vi "Plot Upper & Lower CI Plots.vi"(0 "Y Array":dbl[](array[numeric]), 1 "XY Graph Ref":refnum<vi>, 2 "VI in":refnum<vi>, 3 "Additional LM Data":variant, 5 "X Array":dbl[](array[numeric]), 9 "Weight Array":dbl[](array[numeric]), 11 "error in (no error)":errorcluster, 12 "best fit parameters":dbl[](array[numeric]), 13 "Fitted Plot Name":string, 14 "confidence level (0.68)":dbl=0.68 format="%#_13g") -> (15 "error out":errorcluster)   [LabVIEW 2021, in "Fits.lvlib"]
doc: "Computes the upper and lower confidence interval plots and displays them in the XY Graph."
uses:
  Fits.lvlib
  Graphs/Single Plot Style 2.ctl
  Graphs/Graphs.lvlib
  AlliGator/Decay Analysis/Decay Fit/AlliGator Decay Fit.lvlib
  Graphs/XY Graph/XY Graph Add-Ons.lvlib
panel:
  # "see the License on the block diagram (Ctrl+E or Window:Show Block Diagram)"
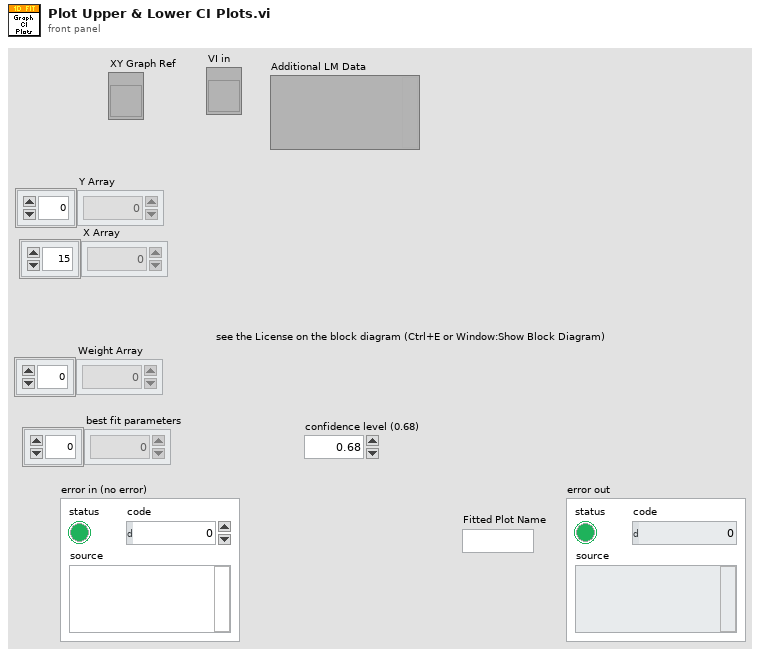
[diagram p1: front panel]
types:
  T1 = typedef "Graphs.lvlib/Single Plot Style 2.ctl" = cluster{"Plot Style":enum16{"unchanged", "Line", "Symbol", "Line + Symbol", "Histogram", "Histogram + Symbol"}, "Histogram Type":enum16{"unchanged", "Left Bound", "Center", "Right Bound"}, "Line Tickness":enum16{"unchanged", "Thin", "1 pixel", "2 pixel", "3 pixel", "4 pixel", "5 pixel"}, "Line Style":enum16{"unchanged", "Plain", "Long Dash", "Short Dash", "Long-Short Dash", "Long-Short-Short Dash"}, "Point Style":enum16{"unchanged", "None", "Empty Circle", "Filled Circle", "Thick Circle", "Dotted Circle", "Empty Square", "Filled Square", "Thick Square", "Dotted Square", "Small Filled Square", "Dot", "Cross", "Tiny Cross", "Large X", "Small x", "Diamond", "Small Empty Square"}, "Line Color":u32, "Line Color defined?":bool, "Point Color":u32, "Point Color defined?":bool, "Anti-aliased":bool}
  T2 = typedef "XY Graph Add-Ons.lvlib/XY Graph Plot Data.ctl" = cluster{"X Array":dbl[], "Y Array":dbl[]}
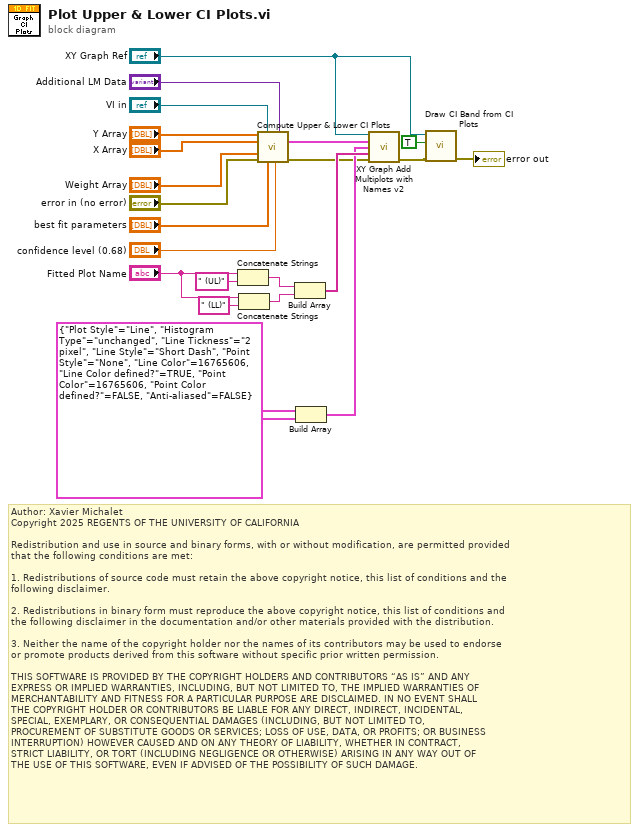
[diagram p0: block diagram]
diagram:
  w15 = T1 {"Plot Style"=enum."Line", "Histogram Type"=enum."unchanged", "Line Tickness"=enum."2 pixel", "Line Style"=enum."Short Dash", "Point Style"=enum."None", "Line Color"=16765606, "Line Color defined?"=TRUE, "Point Color"=16765606, "Point Color defined?"=FALSE, "Anti-aliased"=FALSE} ("Plot Style Array")
  # "Author: Xavier Michalet\nCopyright 2025 REGENTS OF THE UNIVERSITY OF CALIFORNIA\n\nRedistribution and use in source and binary forms, with or without modification, are permitted provided\nthat the following conditions are met:\n\n1. Redistributions of source code must retain the above copyright notice, this list of conditions and the\nfollowing disclaimer.\n\n2. Redistributions in binary form must reproduce the above copyright notice, this list of conditions and\nthe following disclaimer in the documentation and/or other materials provided with the distribution.\n\n3. Neither the name of the copyright holder nor the names of its contributors may be used to endorse \nor promote products derived from this software without specific prior written permission.\n\nTHIS SOFTWARE IS PROVIDED BY THE COPYRIGHT HOLDERS AND CONTRIBUTORS “AS IS” AND ANY \nEXPRESS OR IMPLIED WARRANTIES, INCLUDING, BUT NOT LIMITED TO, THE IMPLIED WARRANTIES OF\nMERCHANTABILITY AND FITNESS FOR A PARTICULAR PURPOSE ARE DISCLAIMED. IN NO EVENT SHALL\nTHE COPYRIGHT HOLDER OR CONTRIBUTORS BE LIABLE FOR ANY DIRECT, INDIRECT, INCIDENTAL, \nSPECIAL, EXEMPLARY, OR CONSEQUENTIAL DAMAGES (INCLUDING, BUT NOT LIMITED TO, \nPROCUREMENT OF SUBSTITUTE GOODS OR SERVICES; LOSS OF USE, DATA, OR PROFITS; OR BUSINESS\nINTERRUPTION) HOWEVER CAUSED AND ON ANY THEORY OF LIABILITY, WHETHER IN CONTRACT, \nSTRICT LIABILITY, OR TORT (INCLUDING NEGLIGENCE OR OTHERWISE) ARISING IN ANY WAY OUT OF\nTHE USE OF THIS SOFTWARE, EVEN IF ADVISED OF THE POSSIBILITY OF SUCH DAMAGE."
  n1 = Concatenate Strings("Fitted Plot Name", " (UL)" ("string")) -> (w19:string)
  n2 = Concatenate Strings("Fitted Plot Name", " (LL)" ("string")) -> (w18:string)
  n3 = call "Compute Upper & Lower CI Plots.vi"("Y Array"="Y Array", "VI in"="VI in", "Additional LM Data"="Additional LM Data", "X Array"="X Array", "Weight Array"="Weight Array", "error in (no error)"="error in (no error)", "best fit parameters"="best fit parameters", "confidence level (0.95)"="confidence level (0.68)") -> ("CI Plots"=w12:T2[], "error out"=w11:errorcluster)  [unwired: 6 in]
  n4 = Build Array(w19, w18) -> (w17:string[])
  n5 = Build Array(w15, w15) -> (w16:T1[])
  n6 = call "XY Graph Add Multiplots with Names v2.vi"("XYGraph in"="XY Graph Ref", "Array of Plots"=w12, "Plots Metadata"=w16, "Array of Plot Names (\"Plot\")"=w17, "error in (no error)"=w11) -> ("error out"=w4:errorcluster)  [unwired: 6 in, 4 out]
  n7 = call "Draw CI Band from CI Plots.vi"("error in (no error)"=w4, "CI Plots?"=TRUE, "XYGraph in"="XY Graph Ref") -> ("error out"=→"error out":errorcluster)  [unwired: 7 in, 1 out]
